vi "Adder.vi"() -> ()   [LabVIEW 2009]
panel:
  out "Result":dbl
  in  "Number 2":dbl
  in  "Number 1":dbl
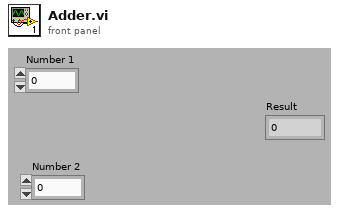
[diagram p1: front panel]
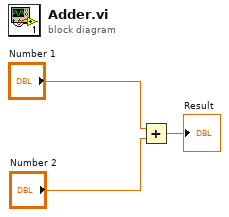
[diagram p0: block diagram]
diagram:
  n1 = Add(x="Number 1", y="Number 2") -> (x+y=→"Result":dbl)
